vi "Decide.vi"(7 "Decide input cluster":T2={"Q Radius"=35, "Threshold"=100, "Compass Bearing"=0.0, "Target Bearing"=0, "Previous Heading"=0, "Raw SICK array"=[], "Camera array "=[], "Calculated bearing vector"={"Numeric"=0.0, "Numeric"=0.0}}) -> (3 "Decide output cluster":T1)   [LabVIEW 2009]
uses:
  Decide output cluster.ctl
panel:
  out "Target Heading":i16
  out "Conv factor":i16
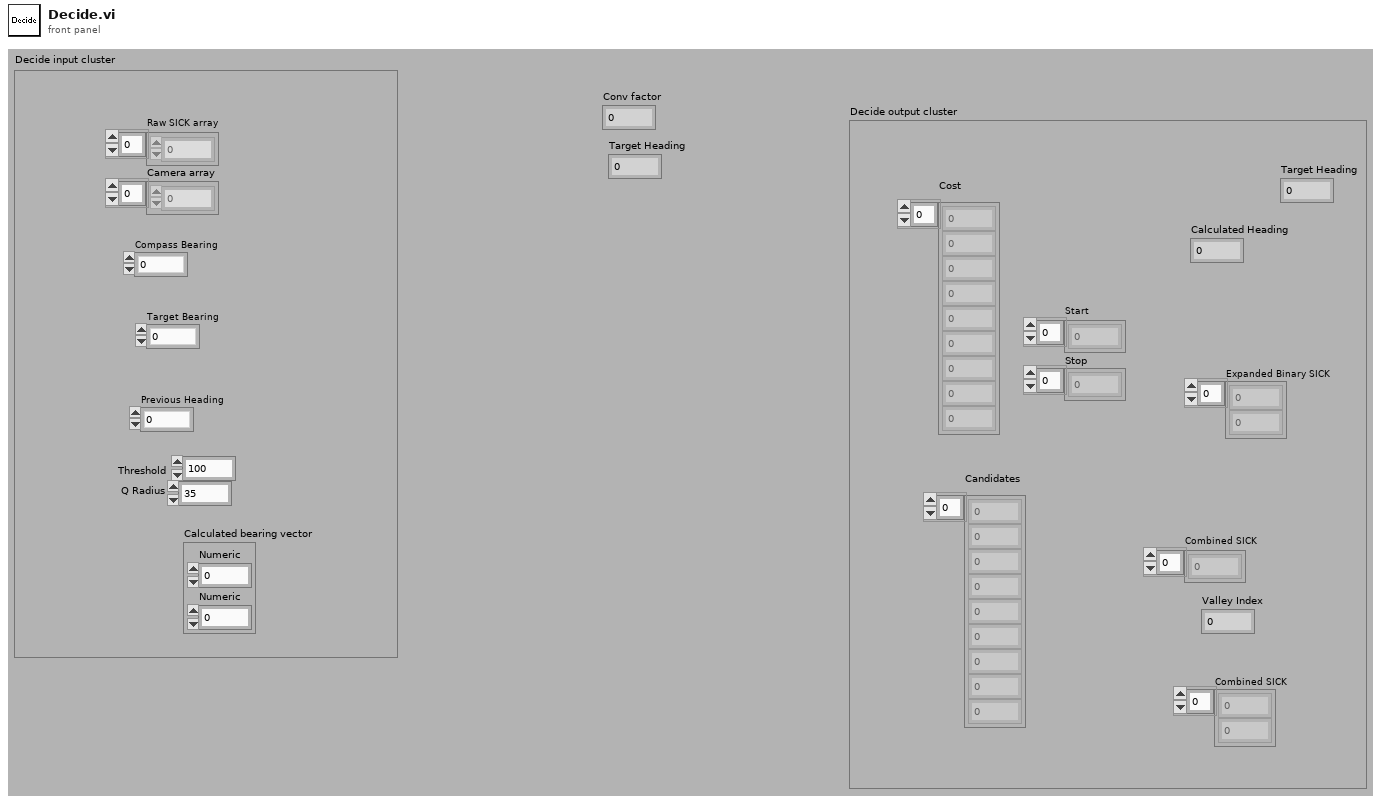
[diagram p1: front panel]
types:
  T1 = typedef "Decide output cluster.ctl" = cluster{"Expanded Binary SICK":i16[], "Target Heading":i16, "Calculated Heading":i16, "Combined SICK":i16[], "Cost":dbl[], "Candidates":i16[], "Start":i16[], "Stop":i16[], "Valley Index":i16, "Combined SICK":i16[]}
  T2 = cluster{"Q Radius":i16, "Threshold":i16, "Compass Bearing":dbl, "Target Bearing":i16, "Previous Heading":i16, "Raw SICK array":i16[], "Camera array ":i16[], "Calculated bearing vector":cluster{"Numeric":dbl, "Numeric":dbl}}
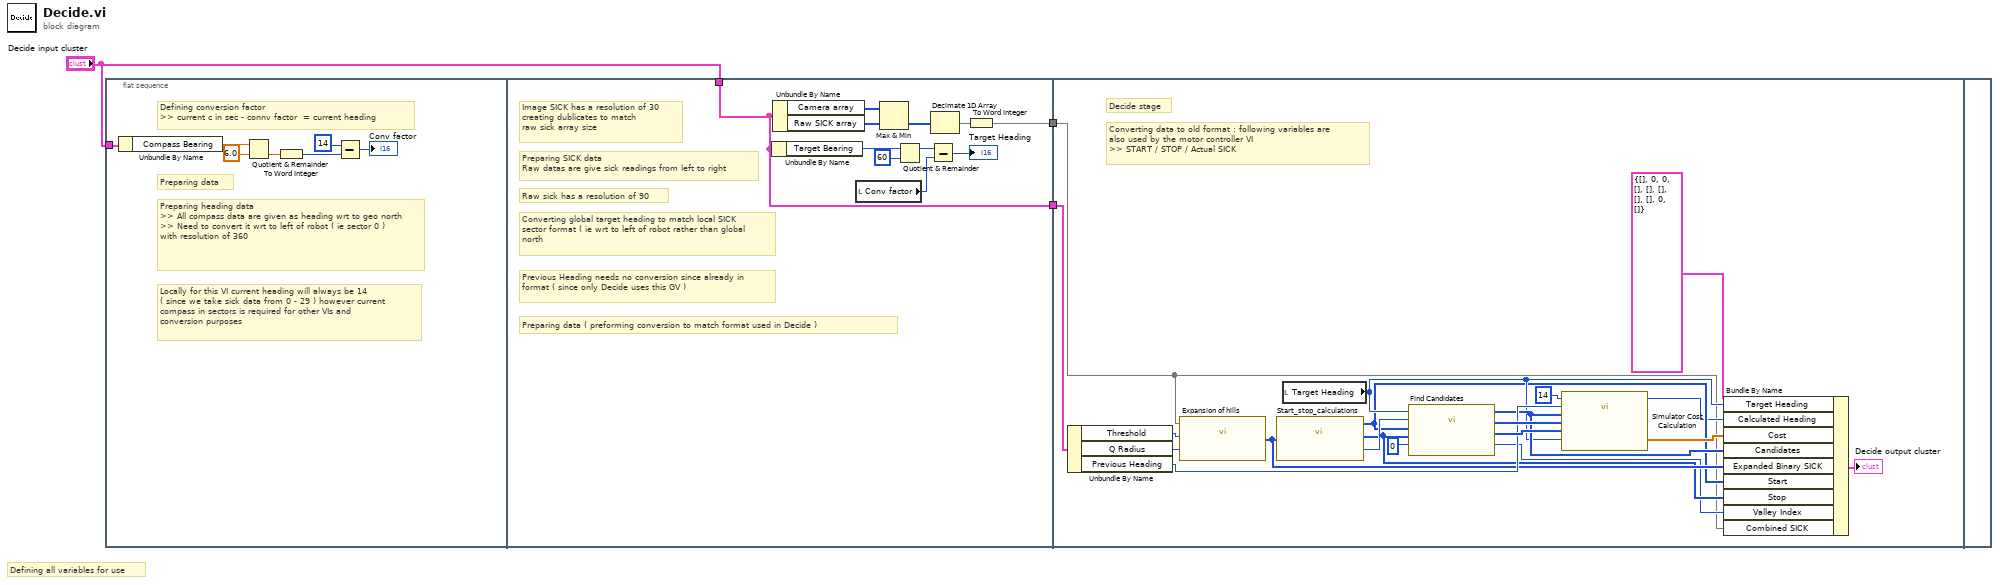
[diagram p0: block diagram]
diagram:
  # "Defining all variables for use"
  n1 = flat-sequence {
    tunnel: "Decide input cluster" -> [w8]
    tunnel: [w16] -> w3
    tunnel: "Decide input cluster" -> [w13]
    tunnel: [w13] -> w1
    tunnel: w3 -> [w22]
    tunnel: w1 -> [w37]
    frame #0 {
      # "Preparing data"
      # "Defining conversion factor\n>> current c in sec - connv factor  = current heading"
      # "Locally for this VI current heading will always be 14\n( since we take sick data from 0 - 29 ) however current \ncompass in sectors is required for other VIs and \nconversion purposes"
      # "Preparing heading data\n>> All compass data are given as heading wrt to geo north\n>> Need to convert it wrt to left of robot ( ie sector 0 )\nwith resolution of 360"
      n2 = Unbundle By Name(w8) -> ("Compass Bearing"=w7:dbl)
      n3 = Quotient & Remainder(x=w7, y=6.0) -> (floor(x/y)=w9:dbl)  [unwired: 1 out]
      n4 = To Word Integer(number=w9) -> (16bit integer=w4:i16)
      n5 = Subtract(x=i16 14, y=w4) -> (x-y=→"Conv factor":i16)
    }
    frame #1 {
      # "Previous Heading needs no conversion since already in format ( since only Decide uses this GV )"
      # "Converting global target heading to match local SICK sector format ( ie wrt to left of robot rather than global north"
      # "Preparing SICK data\nRaw datas are give sick readings from left to right"
      # "Image SICK has a resolution of 30\ncreating dublicates to match \nraw sick array size"
      # "Raw sick has a resolution of 90"
      # "Preparing data ( preforming conversion to match format used in Decide )"
      n6 = Unbundle By Name(w13) -> ("Target Bearing"=w15:i16)
      n7 = Unbundle By Name(w13) -> ("Camera array"=w14:i16[], "Raw SICK array"=w11:i16[])
      n8 = local read "Conv factor"() -> (w20:i16)
      n9 = Max & Min(x=w14, y=w11) -> (min(x,y)=w21:i16[])  [unwired: 1 out]
      n10 = Quotient & Remainder(x=w15, y=i16 60) -> (x-y*floor(x/y)=w19:i16)  [unwired: 1 out]
      n11 = Subtract(x=w19, y=w20) -> (x-y=→"Target Heading":i16)
      n12 = Decimate 1D Array(w21) -> (w17:i16[])  [unwired: 2 out]
      n13 = To Word Integer(number=w17) -> (16bit integer=w16:i16[])
    }
    frame #2 {
      # "Converting data to old format : following variables are\nalso used by the motor controller VI\n>> START / STOP / Actual SICK"
      # "Decide stage"
      n14 = Unbundle By Name(w37) -> ("Threshold"=w36:i16, "Q Radius"=w35:i16, "Previous Heading"=w34:i16)
      n15 = call "Expansion of hills.vi"("Q Radius"=w35, "SICK Threshold"=w36, "Actual SICK"=w22) -> ("Modified Binary SICK"=w32:i16[])
      n16 = call "Start_stop_calculations.vi"("Binary SICK"=w32) -> ("Number of Valleys"=w40:i16, "Stop"=w26:i16[], "Start"=w27:i16[])
      n17 = local read "Target Heading"() -> (w28:i16)
      n18 = call "Find Candidates.vi"("Target Heading"=w28, "Number of Valleys"=w40, "START"=w27, "STOP"=w26, "Expansion delta"=i16 0) -> ("Valley index"=w25:i16, "Candidate Direction"=w30:i16[], "Valley Width"=w39:i16[], "Target Bonus"=w38:i16[])
      n19 = call "Simulator Cost Calculation.vi"("Target Bonus"=w38, "Target Heading"=w28, "Candidate Valley Width"=w39, "Candidates"=w30, "Last Heading"=w34, "Current Heading"=i16 14) -> ("Cost"=w31:dbl[], "Calculated Heading"=w24:i16)
      n20 = Bundle By Name(cluster=T1 {"Expanded Binary SICK"=[], "Target Heading"=0, "Calculated Heading"=0, "Combined SICK"=[], "Cost"=[], "Candidates"=[], "Start"=[], "Stop"=[], "Valley Index"=0, "Combined SICK"=[]} ("Output data cluster"), "Target Heading"=w28, "Calculated Heading"=w24, "Cost"=w31, "Candidates"=w30, "Expanded Binary SICK"=w32, "Start"=w27, "Stop"=w26, "Valley Index"=w25, "Combined SICK"=w22) -> (→"Decide output cluster":T1)
    }
    frame #3 {
    }
  }
